vi "Chirp.vi"() -> ()   [LabVIEW 2019, in "Generator.lvclass"]
uses:
  <vilib>/measure/maUtilsandCtls.llb/ma_Updatet0 timestamp.vi
  Generator.lvclass
  <vilib>/measure/NI_MABase.lvlib
  <vilib>/Analysis/NI_AALBase.lvlib
panel:
  in  "frequency 2":dbl=10.0 format="%0.2p"
  out "Waveform Graph":waveform(dbl)(graph)
  out "phase out":dbl format="%.2p"
  out "signal out":waveform(dbl)
  in  "signal type":T1(ring)
  in  "square wave duty cycle (%)":dbl=50.0 format="%0.2f"
  in  "amplitude":dbl=1.0 format="%0.2p"
  in  "offset":dbl format="%0.2p"
  in  "phase":dbl format="%.2p"
  in  "frequency 1":dbl=10.0 format="%0.2p"
  in  "sampling info":cluster{"Fs":dbl, "#s":dbl}={"Fs"=1000.0, "#s"=1000.0} {"Fs" format="%.2p"}
  in  "reset signal":bool
  out "error out":errorcluster
  in  "error in (no error)":errorcluster
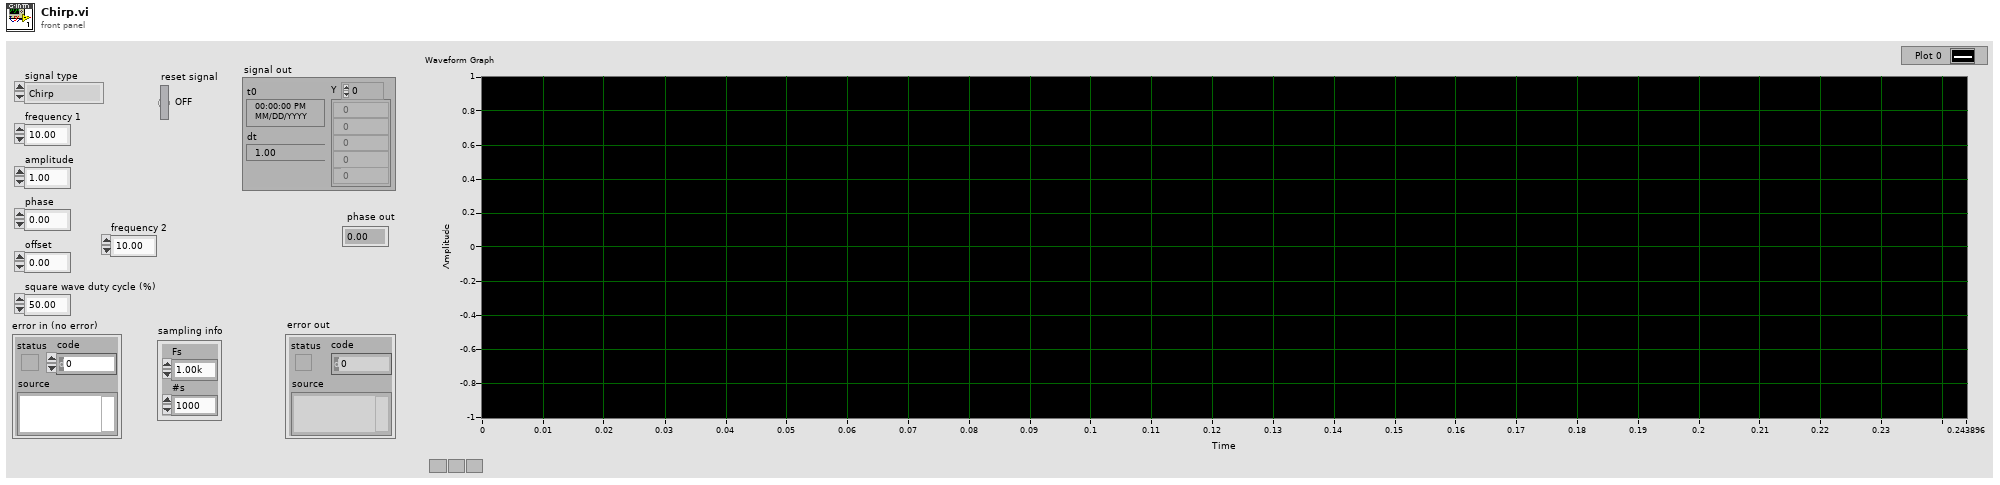
[diagram p1: front panel]
types:
  T1 = enum16{"Chirp", "Triangle Wave", "Square Wave", "Sawtooth Wave"}
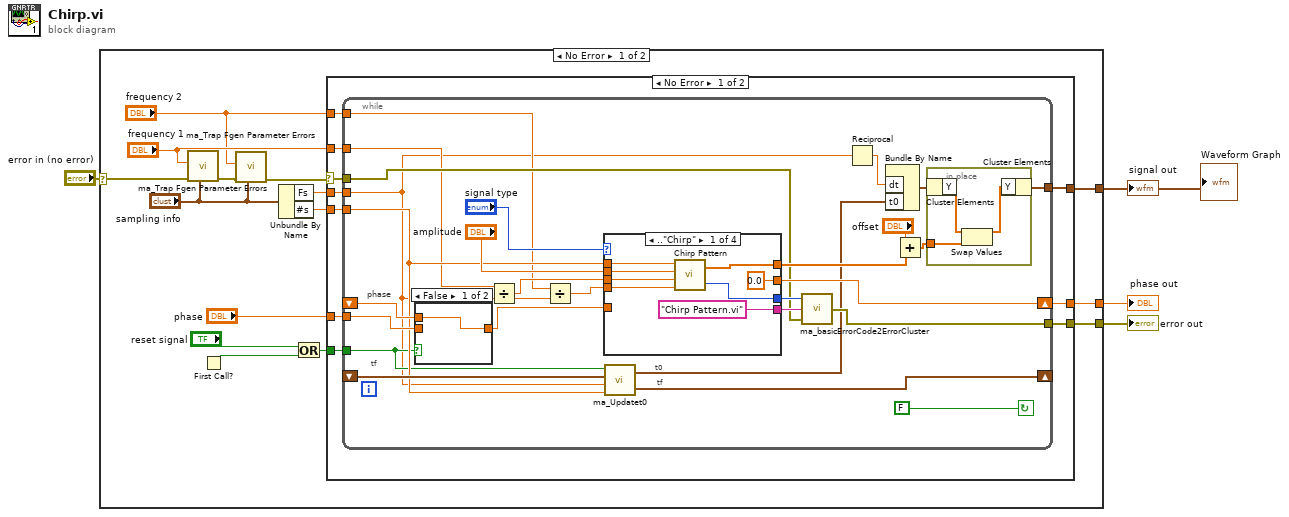
[diagram p0: block diagram]
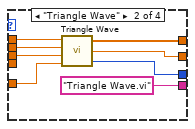
[diagram p2: hidden frame]
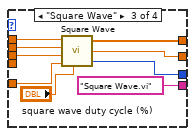
[diagram p3: hidden frame]
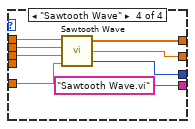
[diagram p4: hidden frame]
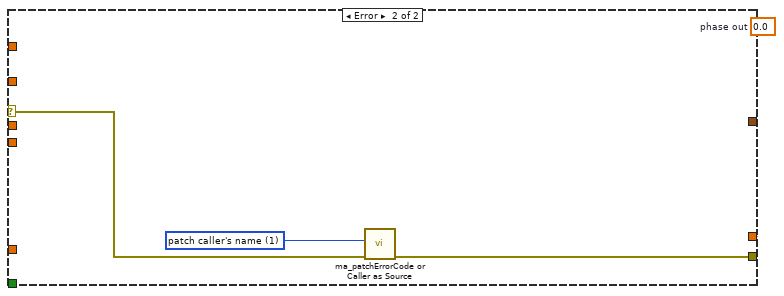
[diagram p6: hidden frame]
diagram:
  n1 = case shown="No Error" "error in (no error)" {
    selector: "error in (no error)" -> [w12 w99]
    tunnel: [w19 w99] -> w4
    tunnel: [w10 _] -> w1
    tunnel: [w9 _] -> w2
    frame No Error {
      n2 = call <vilib>:"ma_Trap Fgen Parameter Errors.vi"("Sampling info"="sampling info", "error in (no error)"=w12, "frequency"="frequency 1") -> ("error out"=w8:errorcluster)  [unwired: 8 in]
      n3 = First Call?() -> (First Call?: T/F=w15:bool)
      n4 = call <vilib>:"ma_Trap Fgen Parameter Errors.vi"("Sampling info"="sampling info", "error in (no error)"=w8, "frequency"="frequency 2") -> ("error out"=w6:errorcluster)  [unwired: 8 in]
      n5 = Unbundle By Name("sampling info") -> ("Fs"=w17:dbl, "#s"=w16:dbl)
      n6 = Or(x="reset signal", y=w15) -> (x .or. y?=w13:bool)
      n7 = case shown="No Error" w6 {
        selector: w6 -> [w23 w97]
        tunnel: [w29 w98] -> w9
        tunnel: [w28 w96] -> w19
        tunnel: "phase" -> [w27 _]
        tunnel: w17 -> [w26 _]
        tunnel: w16 -> [w25 _]
        tunnel: w13 -> [w24 _]
        tunnel: [w21 _] -> w10
        tunnel: "frequency 1" -> [w22 _]
        tunnel: "frequency 2" -> [w20 _]
        frame No Error {
          n8 = while {
            tunnel: w23 -> [w41]
            tunnel: w24 -> [w44]
            tunnel: w25 -> [w45]
            tunnel: w26 -> [w31]
            tunnel: w27 -> [w54]
            tunnel: [w40] -> w28
            shift-left: _ -> [w56]
            shift-right: [w46] -> w29
            shift-left: _ -> [w55]
            shift-right: [w35] -> _
            tunnel: w22 -> [w38]
            tunnel: [w33] -> w21
            tunnel: w20 -> [w32]
            stop <- FALSE continue-if-true
            # "tf"
            # "t0"
            # "phase"
            # "tf"
            n9 = case shown="False" w44 {
              tunnel: w56 -> [w93 _]
              tunnel: [w93 w94] -> w48
              tunnel: w54 -> [_ w94]
              frame False {
              }
              frame True {
              }
            }
            n10 = Divide(x=w38, y=w31) -> (x/y=w51:dbl)
            n11 = Divide(x=w32, y=w31) -> (x/y=w30:dbl)
            n12 = case shown="..\"Chirp\"" "signal type" {
              tunnel: w51 -> [w63 w75 w84 w92]
              tunnel: "amplitude" -> [w64 w74 w83 w91]
              tunnel: w45 -> [w65 w73 w82 w90]
              tunnel: w48 -> [_ w72 w81 w89]
              tunnel: [0.0 ("phase out") w71 w80 w88] -> w46
              tunnel: [w66 w70 w79 w87] -> w50
              tunnel: ["Chirp Pattern.vi" ("subVI Name") "Triangle Wave.vi" ("subVI Name") "Square Wave.vi" ("subVI Name") "Sawtooth Wave.vi" ("subVI Name")] -> w43
              tunnel: [w60 w69 w77 w85] -> w42
              tunnel: w30 -> [w62 _ _ _]
              frame .."Chirp" {
                n13 = call <vilib>:"Chirp Pattern.vi"("f2"=w62, "f1"=w63, "amplitude"=w64, "samples"=w65) -> ("error"=w60:i32, "Chirp Pattern"=w66:dbl[])
              }
              frame "Triangle Wave" {
                n14 = call <vilib>:"Triangle Wave.vi"("samples"=w73, "amplitude"=w74, "frequency"=w75, "phase in"=w72) -> ("triangle wave"=w70:dbl[], "phase out"=w71:dbl, "error"=w69:i32)  [unwired: 1 in]
              }
              frame "Square Wave" {
                n15 = call <vilib>:"Square Wave.vi"("samples"=w82, "amplitude"=w83, "frequency"=w84, "duty cycle (%)"="square wave duty cycle (%)", "phase in"=w81) -> ("square wave"=w79:dbl[], "phase out"=w80:dbl, "error"=w77:i32)  [unwired: 1 in]
              }
              frame "Sawtooth Wave" {
                n16 = call <vilib>:"Sawtooth Wave.vi"("samples"=w90, "amplitude"=w91, "frequency"=w92, "phase in"=w89) -> ("sawtooth wave"=w87:dbl[], "phase out"=w88:dbl, "error"=w85:i32)  [unwired: 1 in]
              }
            }
            n17 = call-poly <vilib>:"ma_Updatet0.vi"("samples"=w45, "sampling rate (S/s)"=w31, "tf previous"=w55, "Reset Generation"=w44) -> ("tf new"=w35:timestamp, "t0"=w39:timestamp)
            n18 = call <vilib>:"ma_basicErrorCode2ErrorCluster.vi"("error in (no error)"=w41, "subVI name"=w43, "Error Code"=w42) -> ("error out"=w40:errorcluster)
            n19 = Reciprocal(x=w31) -> (1/x=w52:dbl)
            n20 = Bundle By Name("dt"=w52, "t0"=w39) -> (w34:waveform(dbl))  [unwired: 1 in]
            n21 = Add(x="offset", y=w50) -> (x+y=w36:dbl[])
            n22 = in-place {
              in-place-border: w36 -> [w57]
              n23 = in-place-cluster #1(w34) -> ("Y"=w59:dbl[])
              n24 = Swap Values(12:w59, 14:w57) -> (1:w58:dbl[])  [unwired: 1 in, 1 out]
              n25 = in-place-cluster #1("Y"=w58) -> (w33:waveform(dbl))
            }
          }
        }
        frame Error {
          w95 = u16 1 items=["patch error code", "patch caller's name"] ("operation")
          w98 = 0.0  # phase out
          n26 = call <vilib>:"ma_patchErrorCode or Caller as Source.vi"("error in (no error)"=w97, "operation"=w95) -> ("error out"=w96:errorcluster)  [unwired: 9 in]
        }
      }
    }
    frame Error {
    }
  }
  "error out" <- w4
  "signal out" <- w1
  "phase out" <- w2
  "Waveform Graph" <- w1
